vi "Handle Error.vi"(8 "error in (no error)":errorcluster, 11 "GenNet Protocol in":refnum<class "GenNet Protocol.lvclass">) -> (0 "error out":errorcluster, 1 "Add Info for Error Broadcast":string, 2 "Module ID for Error Broadcast":i32=-1, 3 "GenNet Protocol out":refnum<class "GenNet Protocol.lvclass">)   [LabVIEW 2022 SP3, in "hse-gennet.lvlib" / "GenNet Protocol.lvclass"]
doc: "____\nHAMPEL SOFTWARE ENGINEERING v3.8.0 (2023-12-18 14:41)"
uses:
  GenNet Protocol.lvclass
  GenNet Protocol.lvclass/GenNet Protocol.ctl
  Get Module ID.vi
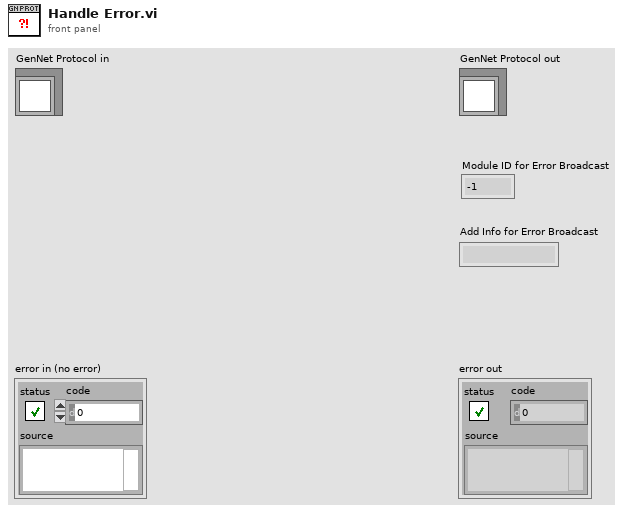
[diagram p1: front panel]
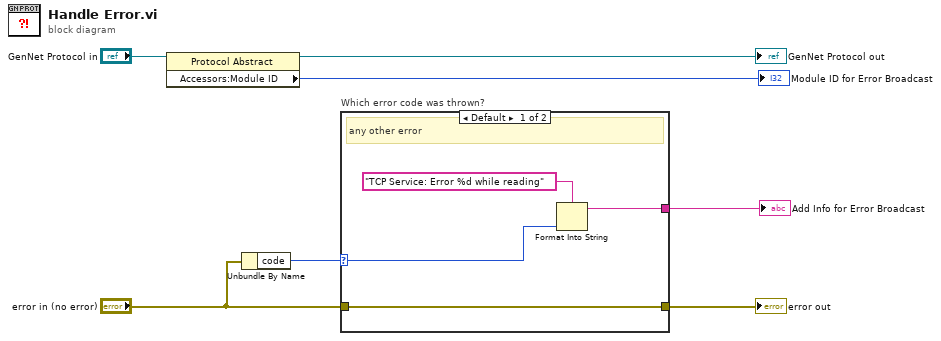
[diagram p0: block diagram]
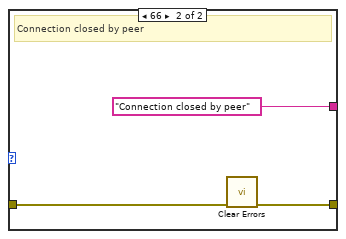
[diagram p2: hidden frame]
diagram:
  n1 = property class="Protocol Abstract"(reference="GenNet Protocol in") -> (reference out=→"GenNet Protocol out":refnum<class "GenNet Protocol.lvclass">, "Accessors:Module ID"=→"Module ID for Error Broadcast":i32)  [unwired: 1 in, 1 out]
  n2 = Unbundle By Name("error in (no error)") -> ("code"=w7:i32)
  n3 = case "Which error code was thrown?" shown="Default" w7 {
    selector: w7 -> [w8 _]
    tunnel: "error in (no error)" -> [w11 w13]
    tunnel: [w11 w12] -> w2
    tunnel: [w9 "Connection closed by peer" ("format string")] -> w3
    frame Default {
      # "any other error"
      n4 = Format Into String(format string="TCP Service: Error %d while reading" ("Additional Information"), w8) -> (resulting string=w9:string)  [unwired: 2 in, 1 out]
    }
    frame 66 {
      # "Connection closed by peer"
      n5 = call <vilib>:"Clear Errors.vi"("error in (no error)"=w13) -> ("error out"=w12:errorcluster)  [unwired: 5 in, 1 out]
    }
  }
  "error out" <- w2
  "Add Info for Error Broadcast" <- w3
